vi "Write I16.vi"(7 "RegisterOffset":u32, 8 "error in":errorcluster, 9 "value in":i16, 10 "register name":string, 11 "session in":u32) -> (0 "error out":errorcluster, 3 "session out":u32)   [LabVIEW 2020, in "FPGA Register IO.lvlib"]
uses:
  FPGA Register IO.lvlib
  NiFpga.dll
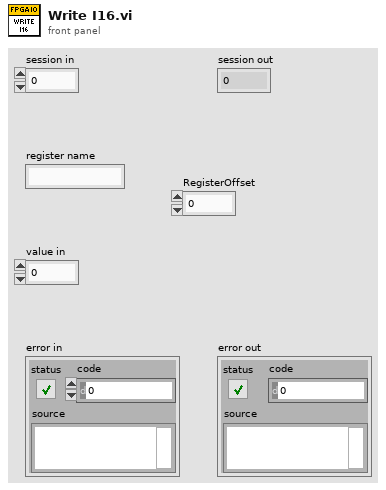
[diagram p1: front panel]
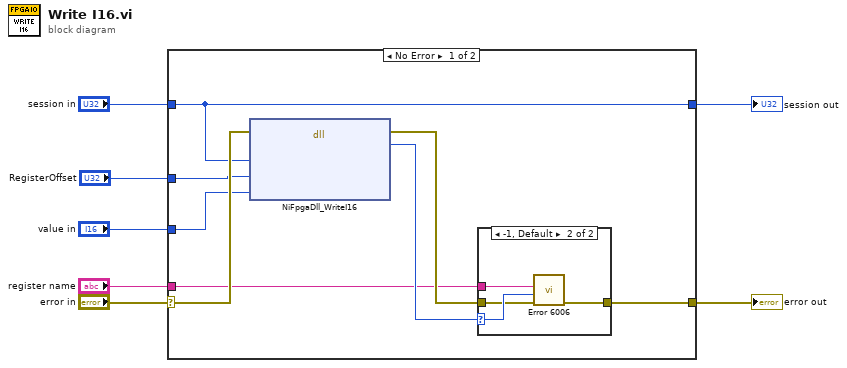
[diagram p0: block diagram]
diagram:
  n1 = case shown="No Error" "error in" {
    selector: "error in" -> [w15 w22]
    tunnel: "session in" -> [w14 w21]
    tunnel: [w9 w22] -> w6
    tunnel: [w14 w21] -> w5
    tunnel: "value in" -> [w13 _]
    tunnel: "register name" -> [w10 _]
    tunnel: "RegisterOffset" -> [w8 _]
    frame No Error {
      n2 = dll-call lib="NiFpga.*" fn="NiFpgaDll_WriteI16"(error in=w15, "session"=w14, "offset"=w8, "value"=w13) -> (error out=w12:errorcluster, "status"=w11:i32)  [unwired: 5 in, 1 out]
      n3 = case shown="-1, Default" w11 {
        selector: w11 -> [_ w18]
        tunnel: w12 -> [w16 w17]
        tunnel: [w16 w20] -> w9
        tunnel: w10 -> [_ w19]
        frame 0 {
        }
        frame -1, Default {
          n4 = call "Error 6006.vi"("error in (no error)"=w17, "rio status code"=w18, "register name"=w19) -> ("error out"=w20:errorcluster)  [unwired: 8 in]
        }
      }
    }
    frame Error {
    }
  }
  "error out" <- w6
  "session out" <- w5
